vi "Breakdown Rep.vi"() -> ()   [LabVIEW 2017]
panel:
  out "Breakdown Report":bool
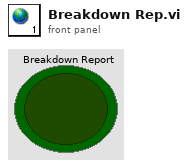
[diagram p1: front panel]
diagram:
